vi "Test PINGREQ packet.vi"() -> ()   [LabVIEW 2013]
uses:
  Control Packets/PINGREC/PINGREC.lvclass
  Control Packets/ControlPacket/ControlPacket.lvclass/ControlPacket.ctl
  Control Packets/ControlPacket/ControlPacket.lvclass
panel:
  out "Packet ID":u16 format="%04x"
  out "error out":errorcluster
  out "Absence of Packet Identifier":bool
  out "Packet type":bool
  out "All packets consumed":bool
  out "Complete Packet":bool
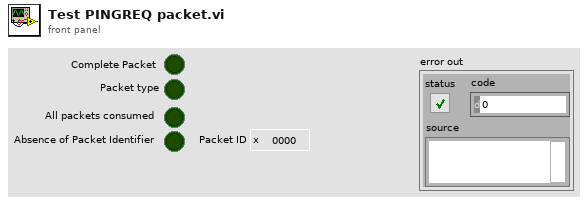
[diagram p1: front panel]
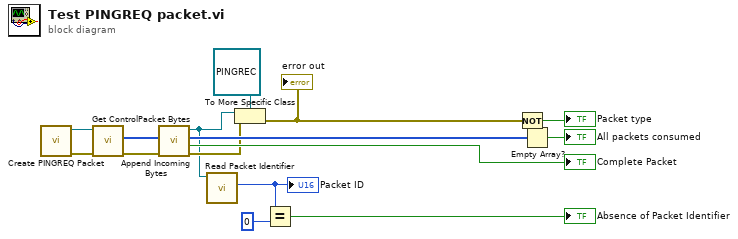
[diagram p0: block diagram]
diagram:
  n1 = call "Create PINGREQ Packet.vi"() -> ("error out"=w1:errorcluster, "PINGREC out"=w3:refnum<class "PINGREC.lvclass">)  [unwired: 10 in]
  n2 = call "Get ControlPacket Bytes.vi"("error in (no error)"=w1, "ControlPacket"=w3) -> ("error out"=w9:errorcluster, "Bytes Stream"=w15:u8[])  [unwired: 7 in, 1 out]
  n3 = call "Append Incoming Bytes.vi"("error in (no error)"=w9, "Incoming Packets"=w15) -> ("error out"=w8:errorcluster, "Complete Packet"=→"Complete Packet":bool, "Remaining Packets"=w13:u8[], "ControlPacket"=w5:refnum<class "ControlPacket.lvclass">)  [unwired: 6 in]
  n4 = call "Read Packet Identifier.vi"("ControlPacket in"=w5) -> ("Packet Identifier"=w7:u16)  [unwired: 9 in, 1 out]
  "Packet ID" <- w7
  n5 = To More Specific Class(target class=refnum<class "PINGREC.lvclass"> refnum ("PINGREC.lvclass"), reference=w5, error in=w8) -> (error out=w11:errorcluster)  [unwired: 1 out]
  "error out" <- w11
  n6 = Equal?(x=w7, y=u16 0) -> (x = y?=→"Absence of Packet Identifier":bool)
  n7 = Not(x=w11) -> (.not. x?=→"Packet type":bool)
  n8 = Empty Array?(array=w13) -> (empty?=→"All packets consumed":bool)
